vi "Read Status Byte Query.vi"(0 "VISA resource name":refnum<visa-resource-name>, 11 "error in (no error)":errorcluster) -> (4 "VISA resource name out":refnum<visa-resource-name>, 6 "Status Byte Register":T1, 15 "error out":errorcluster)   [LabVIEW 2014, in "Associated Power Technologies 8500 Series.lvlib"]
doc: "Queries the <B>Status Byte</B>. Returns the decimal value of the binary-weighted sum of bits.\n\nEach bit represents a status in the instrument.\n\nEx : When Test passes, BIT 0 is set High giving status \"ALL PASS\"\n\nBIT 0 ,01H,(1) All PASS\nBIT 1 ,02H,(2) FAIL\nBIT 2, 04H,(4) ABORT\nBIT 3, 08H,(8) Process\nBIT 4, 10H,(16) Message Available\nBIT 5, 20H,(32) Standard Event (ESB)\nBIT 6, 40H,(64) Request Service (MSS)\nBIT 7, 80H,(128) Prompt"
uses:
  <instrlib>/Associated Power Technologies 8500 Series/Associated Power Technologies 8500 Series.lvlib
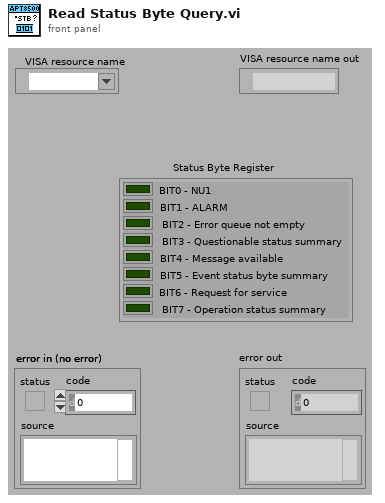
[diagram p1: front panel]
types:
  T1 = cluster{"BIT0 - NU1":bool, "BIT1 - ALARM":bool, "BIT2 - Error queue not empty":bool, "BIT3 - Questionable status summary":bool, "BIT4 - Message available":bool, "BIT5 - Event status byte summary":bool, "BIT6 - Request for service":bool, "BIT7 - Operation status summary":bool}
  T2 = cluster{"Boolean array[0]":bool, "Boolean array[1]":bool, "Boolean array[2]":bool, "Boolean array[3]":bool, "Boolean array[4]":bool, "Boolean array[5]":bool, "Boolean array[6]":bool, "Boolean array[7]":bool}
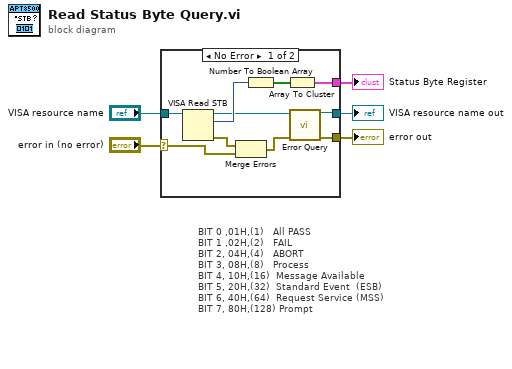
[diagram p0: block diagram]
diagram:
  # "BIT 0 ,01H,(1)   All PASS\nBIT 1 ,02H,(2)   FAIL\nBIT 2, 04H,(4)   ABORT\nBIT 3, 08H,(8)   Process\nBIT 4, 10H,(16)  Message Available\nBIT 5, 20H,(32)  Standard Event  (ESB)\nBIT 6, 40H,(64)  Request Service (MSS)\nBIT 7, 80H,(128) Prompt"
  n1 = case shown="No Error" "error in (no error)" {
    selector: "error in (no error)" -> [w6 w16]
    tunnel: [w15 _] -> w5
    tunnel: "VISA resource name" -> [w14 w17]
    tunnel: [w13 w17] -> w3
    tunnel: [w12 w16] -> w2
    frame No Error {
      n2 = VISA Read STB(11:w14) -> (0:w8:errorcluster, 2:w11:u16, 3:w9:refnum<visa-resource-name>)  [unwired: 1 in]
      n3 = Merge Errors(w8, w6) -> (w7:errorcluster)
      n4 = Number To Boolean Array(number=w11) -> (Boolean array=w10:bool[])
      n5 = Array To Cluster(array=w10) -> (cluster=w15:T2)
      n6 = call <instrlib>:"Error Query.vi"("VISA resource name"=w9, "error in (no error)"=w7) -> ("VISA resource name out"=w13:refnum<visa-resource-name>, "error out"=w12:errorcluster)  [unwired: 10 in, 2 out]
    }
    frame Error {
    }
  }
  "Status Byte Register" <- w5
  "VISA resource name out" <- w3
  "error out" <- w2
